vi "brightSpotThreshold.vi"(8 "error in (no error)":errorcluster, 10 "mintemp":dbl, 11 "ax5 in":refnum<class "ax5.lvclass">) -> (0 "error out":errorcluster, 1 "sglImage":T1, 2 "clippedTemperature":sgl[][](array[numeric]), 3 "ax5 out":refnum<class "ax5.lvclass">)   [LabVIEW 2017, in "ax5.lvclass"]
uses:
  ax5.lvclass
  <vilib>/vision/Image Controls.llb/IMAQ Image.ctl
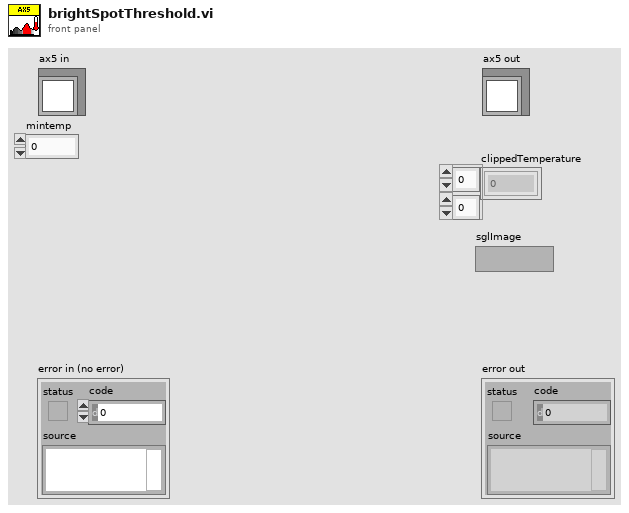
[diagram p1: front panel]
types:
  T1 = typedef "IMAQ Image.ctl" = refnum<image>
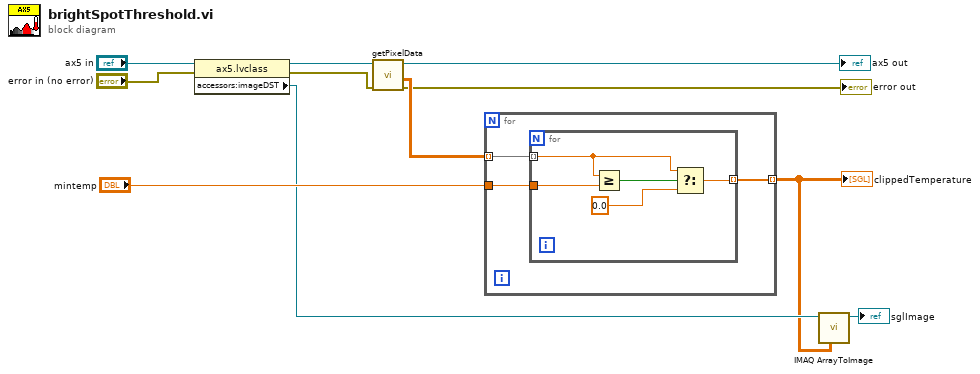
[diagram p0: block diagram]
diagram:
  n1 = property class="ax5.lvclass"(reference="ax5 in", error in="error in (no error)") -> (reference out=w10:refnum<class "ax5.lvclass">, error out=w9:errorcluster, "accessors:imageDST"=w3:T1)
  n2 = call-dynamic "getPixelData.vi"("error in (no error)"=w9, "ax5 in"=w10) -> ("error out"=→"error out":errorcluster, "Temp"=w6:dbl[][], "ax5 out"=→"ax5 out":refnum<class "ax5.lvclass">)  [unwired: 5 in, 2 out]
  n3 = for {
    tunnel: w6 -> [w14] mode=indexing
    tunnel: "mintemp" -> [w13]
    tunnel: [w12] -> w2 mode=indexing
    n4 = for {
      tunnel: w14 -> [w17] mode=indexing
      tunnel: w13 -> [w19]
      tunnel: [w15] -> w12 mode=indexing
      n5 = Greater Or Equal?(x=w17, y=w19) -> (x >= y?=w18:bool)
      n6 = Select(t=w17, s=w18, f=0.0) -> (s? t:f=w15:dbl)
    }
  }
  "clippedTemperature" <- w2
  n7 = call "IMAQ ArrayToImage"("Image Pixels (Float)"=w2, "Image"=w3) -> ("Image Out"=→"sglImage":T1)  [unwired: 8 in, 1 out]
